vi "Rename DAQmx Devices Based on Serial Number.vi"(0 "Serial Numbers":string[](array[string]), 5 "New DAQmx Names":string[](array[string]), 11 "Error In":errorcluster) -> (15 "Error Out":errorcluster)   [LabVIEW 2016]
uses:
  <vilib>/nisyscfg/Initialize (Control).vi
  <vilib>/nisyscfg/Find Hardware.vi
  <vilib>/nisyscfg/Close (Hardware).vi
  <vilib>/nisyscfg/Close (System).vi
  <vilib>/nisyscfg/nisyscfg.lvlib
  <resource>/objmgr/nisysapi.rc
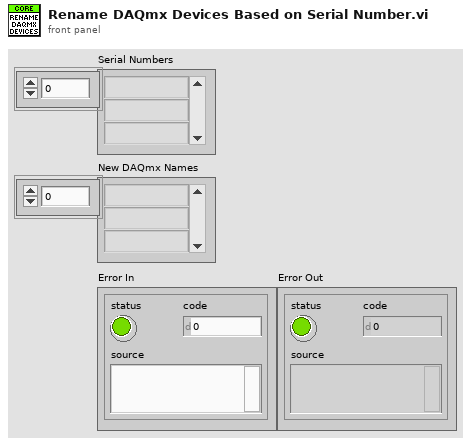
[diagram p1: front panel]
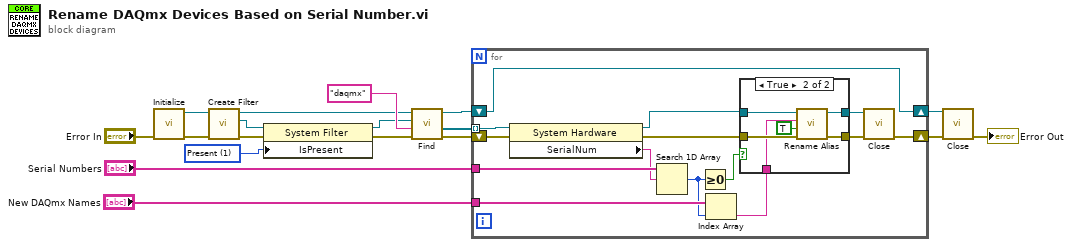
[diagram p0: block diagram]
diagram:
  w5 = 1 items=["Unknown"=-1, "Not Present"=0, "Present"=1] ("Is Present")
  n1 = call-poly <vilib>:"Initialize.vi"("error in (no error)"="Error In") -> ("error out"=w11:errorcluster, "Session out"=w12:refnum<k21>)  [unwired: 8 in, 1 out]
  n2 = call <vilib>:"Create Filter.vi"("error in (no error)"=w11, "Session in"=w12) -> ("error out"=w9:errorcluster, "Filter out"=w10:refnum<k20>, "Session out"=w8:refnum<k21>)  [unwired: 7 in]
  n3 = property class="System Filter"(reference=w10, error in=w9, "IsPresent"=w5) -> (reference out=w6:refnum<k20>, error out=w7:errorcluster)
  n4 = call-poly <vilib>:"Find.vi"("error in (no error)"=w7, "Experts"="daqmx" ("experts"), "Filter in"=w6, "Session in"=w8) -> ("error out"=w13:errorcluster, "Resources out"=w17:refnum<k20>[], "Session out"=w16:refnum<k21>)  [unwired: 4 in, 1 out]
  n5 = for {
    tunnel: w17 -> [w32] mode=indexing
    tunnel: "Serial Numbers" -> [w27]
    tunnel: "New DAQmx Names" -> [w24]
    shift-right: [w31] -> w15
    shift-left: w16 -> [w31]
    shift-right: [w20] -> w14
    shift-left: w13 -> [w30]
    n6 = property class="System Hardware"(reference=w32, error in=w30) -> (reference out=w29:refnum<k20>, error out=w28:errorcluster, "SerialNum"=w26:string)
    n7 = Search 1D Array(1D array=w27, element=w26) -> (index of element=w23:i32)  [unwired: 1 in]
    n8 = Greater Or Equal To 0?(x=w23) -> (x >= 0?=w25:bool)
    n9 = Index Array(array=w24, index=w23) -> (element=w22:string)
    n10 = case shown="True" w25 {
      tunnel: w29 -> [w33 w40]
      tunnel: w28 -> [w34 w39]
      tunnel: [w34 w36] -> w21
      tunnel: w22 -> [_ w37]
      tunnel: [w33 w35] -> w19
      frame False {
      }
      frame True {
        n11 = call <vilib>:"Rename Alias.vi"("error in (no error)"=w39, "Overwrite Conflict (F)"=TRUE ("overwrite (F)"), "New Name"=w37, "Resource in"=w40) -> ("error out"=w36:errorcluster, "Resource out"=w35:refnum<k20>)  [unwired: 4 in, 2 out]
      }
    }
    n12 = call-poly <vilib>:"Close.vi"("error in (no error)"=w21, "Resource in"=w19) -> ("error out"=w20:errorcluster)  [unwired: 9 in]
  }
  n13 = call-poly <vilib>:"Close.vi"("error in (no error)"=w14, "Session in"=w15) -> ("error out"=→"Error Out":errorcluster)  [unwired: 9 in]
